vi "SpecAn Calibrate Set.vi"(8 "error in (no error)":errorcluster, 11 "VISA resource name":refnum<visa-resource-name>) -> (0 "error out":errorcluster, 1 "Self-Test Result Message":string, 2 "Self-Test Result Code":i32, 3 "VISA resource name out":refnum<visa-resource-name>)   [LabVIEW 2015]
doc: "Runs the instrument's self-test routine and returns the test results."
uses:
  Controls/FGV Action SpecAn Model.ctl
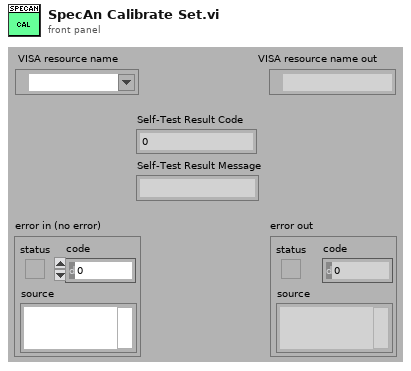
[diagram p1: front panel]
types:
  T1 = typedef "FGV Action SpecAn Model.ctl" = enum16{"Get", "Set"}
  T2 = typedef "SpecAn Model.ctl" = enum16{"E4440", "N9030"}
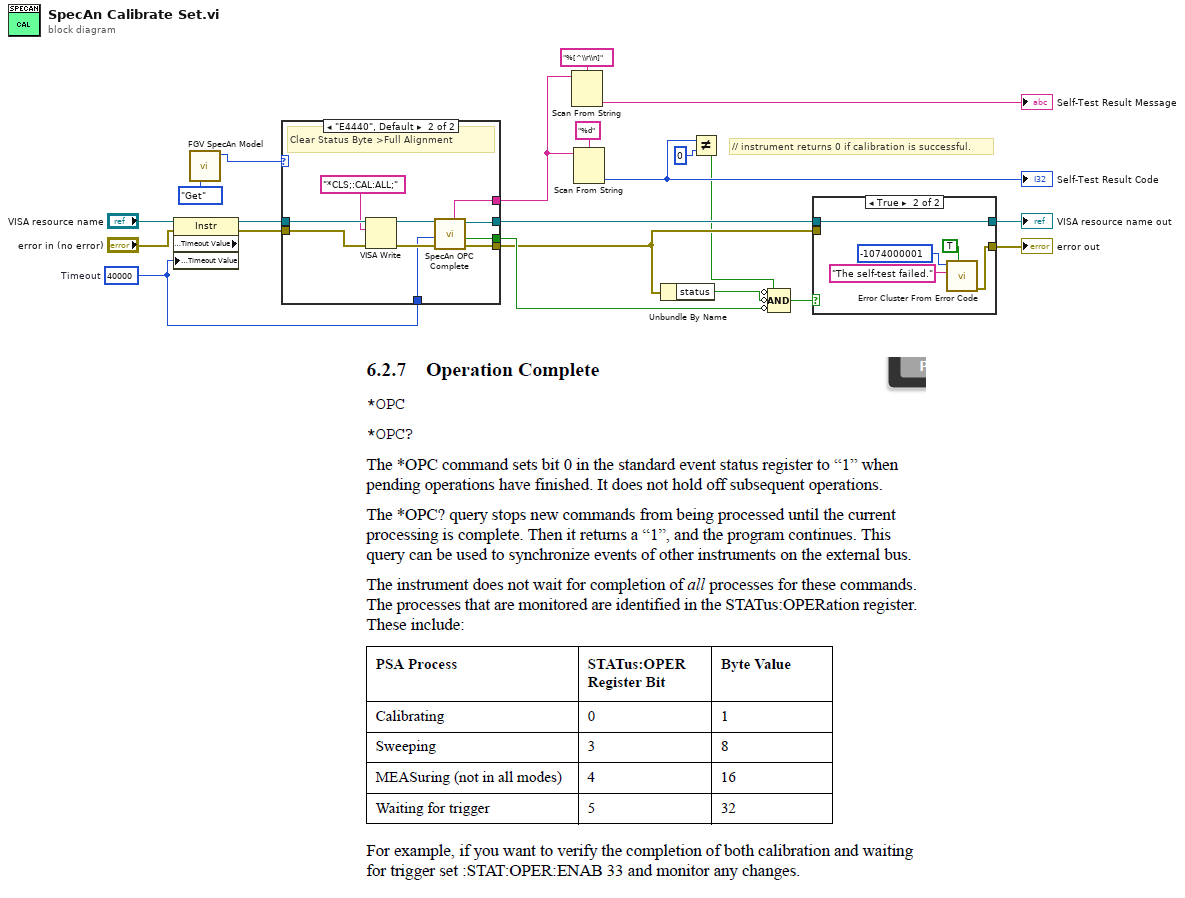
[diagram p0: block diagram]
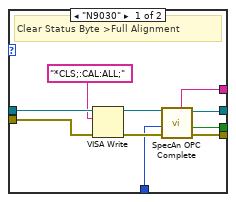
[diagram p2: hidden frame]
diagram:
  w10 = u32 40000  # Timeout
  # "// instrument returns 0 if calibration is successful."
  n1 = property class="Instr" props=["General Settings:Timeout Value", "General Settings:Timeout Value"](reference="VISA resource name", error in="error in (no error)", "General Settings:Timeout Value"=w10) -> (reference out=w15:refnum<visa-resource-name>, error out=w16:errorcluster)  [unwired: 1 out]
  n2 = call "FGV SpecAn Model.vi"("Action"=FGV_Action_SpecAn_Model."Get") -> ("SA Model"=w8:T2)  [unwired: 6 in, 1 out]
  n3 = case shown="\"E4440\", Default" w8 {
    tunnel: w16 -> [w31 w41]
    tunnel: w15 -> [w30 w40]
    tunnel: w10 -> [w25 w35]
    tunnel: [w24 w34] -> w2
    tunnel: [w27 w37] -> w3
    tunnel: [w23 w33] -> w5
    tunnel: [w22 w32] -> w4
    frame "N9030" {
      # "Clear Status Byte >Full Alignment"
      n4 = VISA Write(VISA resource name=w30, write buffer="*CLS;:CAL:ALL;" ("Set Full Alignment"), error in (no error)=w31) -> (VISA resource name out=w26:refnum<visa-resource-name>, error out=w28:errorcluster)  [unwired: 1 out]
      n5 = call "SpecAn OPC Complete.vi"("Error In"=w28, "Max Time (ms)"=w25, "VISA In"=w26) -> ("Error Out"=w27:errorcluster, "TimedOut"=w23:bool, "VISA Out"=w24:refnum<visa-resource-name>, "StatusByte"=w22:string)  [unwired: 4 in, 1 out]
    }
    frame "E4440", Default {
      # "Clear Status Byte >Full Alignment"
      n6 = VISA Write(VISA resource name=w40, write buffer="*CLS;:CAL:ALL;" ("Set Full Alignment"), error in (no error)=w41) -> (VISA resource name out=w36:refnum<visa-resource-name>, error out=w38:errorcluster)  [unwired: 1 out]
      n7 = call "SpecAn OPC Complete.vi"("Error In"=w38, "Max Time (ms)"=w35, "VISA In"=w36) -> ("Error Out"=w37:errorcluster, "TimedOut"=w33:bool, "VISA Out"=w34:refnum<visa-resource-name>, "StatusByte"=w32:string)  [unwired: 4 in, 1 out]
    }
  }
  n8 = Scan From String(format string="%[^\\r\\n]" ("Format String"), input string=w4) -> (output 1=→"Self-Test Result Message":string)  [unwired: 3 in, 3 out]
  n9 = Scan From String(format string="%d", input string=w4) -> (output 1=w12:i32)  [unwired: 3 in, 3 out]
  "Self-Test Result Code" <- w12
  n10 = Unbundle By Name(w3) -> ("status"=w14:bool)
  n11 = Not Equal?(x=w12, y=0) -> (x != y?=w1:bool)
  n12 = Compound Arithmetic op=AND(invert w1, invert w14, invert w5) -> (w13:bool)
  n13 = case shown="True" w13 {
    tunnel: w2 -> [w43 w48]
    tunnel: w3 -> [w42 _]
    tunnel: [w42 w44] -> w7
    tunnel: [w43 w48] -> w6
    frame False {
    }
    frame True {
      n14 = call <vilib>:"Error Cluster From Error Code.vi"("show call chain? (False)"=TRUE, "error message (\"\")"="The self-test failed." ("Source (VI Name)"), "error code (0)"=-1074000001 ("Code")) -> ("error out"=w44:errorcluster)  [unwired: 6 in]
    }
  }
  "VISA resource name out" <- w6
  "error out" <- w7
